vi "test.flatten.ClusterCfgTable.vi"() -> ()   [LabVIEW 2017]
uses:
  Configuration/ClusterCfgTable/ClusterCfgTable.lvlib
panel:
  out "ConfigStrings":string[](array[string])
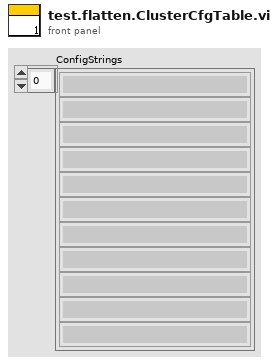
[diagram p1: front panel]
types:
  T1 = cluster{"Direction":enum16{"Input - 输入", "Output - 输出", "Record - 记录"}, "Group":string, "Name":string, "ID":string, "DataType":enum16{"0 ___ 没有使用通道", "1 ___ BOOLEAN", "2 ___ U16", "3 ___ DBL"}, "Protocol":string, "Description":string}
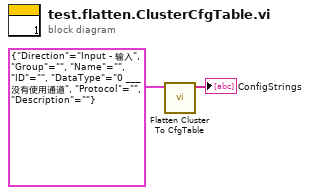
[diagram p0: block diagram]
diagram:
  n1 = call "Flatten Cluster To CfgTable.vi"("Cluster Configuration Typedef"=T1 {"Direction"=enum."Input - 输入", "Group"="", "Name"="", "ID"="", "DataType"=enum."0 ___ 没有使用通道", "Protocol"="", "Description"=""} ("PhyChannelCfg")) -> ("CfgTable Row"=→"ConfigStrings":string[])  [unwired: 9 in, 1 out]
